vi "flashcard draw ui.vi"(0 "Color":refnum<vi>, 1 "stop":refnum<vi>, 2 "Array Info":u16[][](array[ring]) items=["Black", "White", "Orange", "Red", "Blue", "Green", "Disabled"], 3 "Cursor Size":refnum<vi>, 4 "Stunt":refnum<vi>, 5 "Flashcard Array":refnum<vi>) -> ()   [LabVIEW 2019, in "flashcards.lvlib"]
uses:
  flashcards.lvlib
  flashcards.llb/ctl_flashcard.ctl
  Colors.ctl
panel:
  in  "Pic Ring":T1
  in  "stop":bool
  out "Array":T1[][](array[typedef])=[[0, 0, 0, 0, 0, 0, 0, 0, 0, 0, 0], [0, 0, 0, 0, 0, 0, 0, 0, 0, 0, 0], [0, 0, 0, 0, 0, 0, 0, 0, 0, 0, 0], [0, 0, 0, 0, 0, 0, 0, 0, 0, 0, 0], [0, 0, 0, 0, 0, 0, 0, 0, 0, 0, 0], [0, 0, 0, 0, 0, 0, 0, 0, 0, 0, 0], [0, 0, 0, 0, 0, 0, 0, 0, 0, 0, 0], [0, 0, 0, 0, 0, 0, 0, 0, 0, 0, 0], [0, 0, 0, 0, 0, 0, 0, 0, 0, 0, 0], [0, 0, 0, 0, 0, 0, 0, 0, 0, 0, 0], [0, 0, 0, 0, 0, 0, 0, 0, 0, 0, 2]]
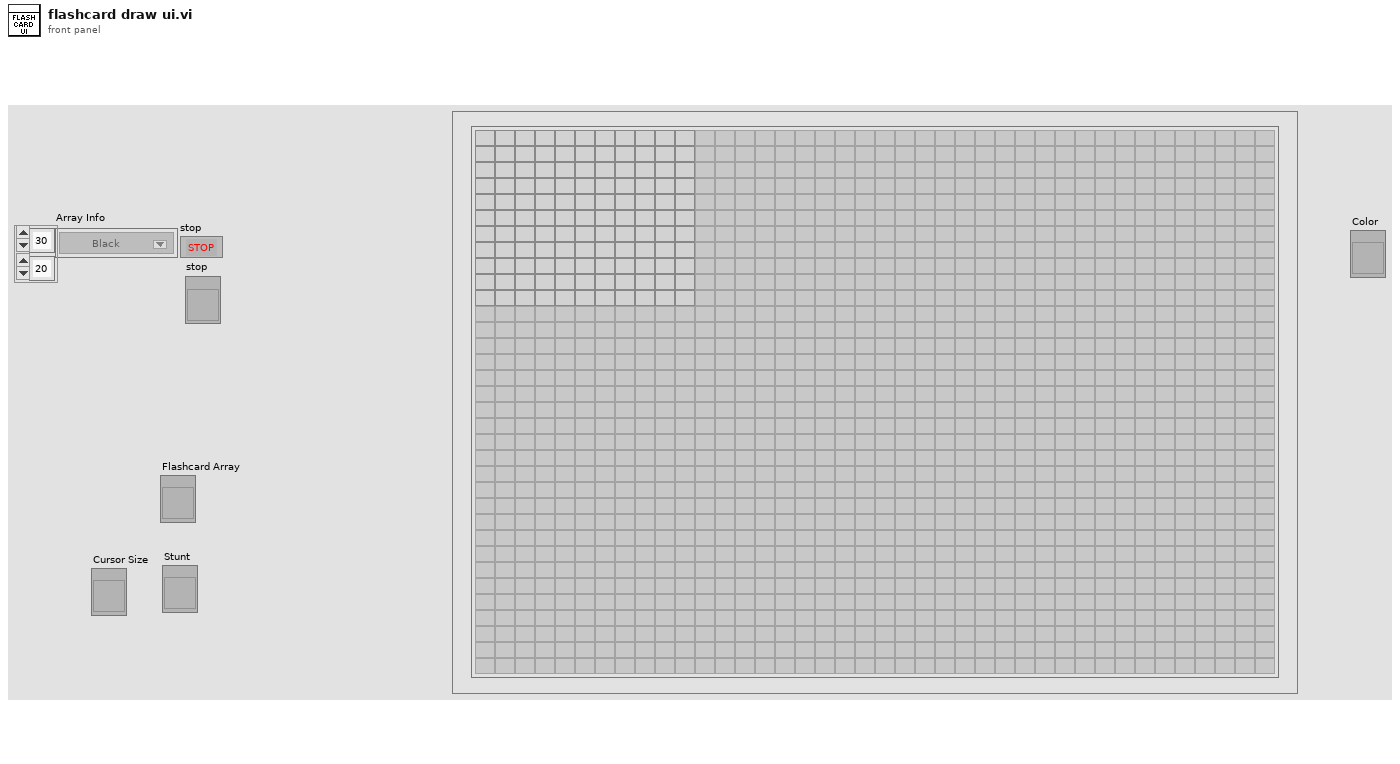
[diagram p1: front panel]
types:
  T1 = typedef "flashcards.lvlib/ctl_flashcard.ctl" = u16
  T2 = typedef "LVPositionTypeDef.ctl" = cluster{"Left":i32, "Top":i32}
  T3 = typedef "LVBoundsTypeDef.ctl" = cluster{"Width":u32, "Height":u32}
  T4 = typedef "LVPoint32TypeDef.ctl" = cluster{"Horizontal":i32, "Vertical":i32}
  T5 = typedef "Colors.ctl" = enum16{"Black", "White", "Orange", "Red", "Blue", "Green", "None"}
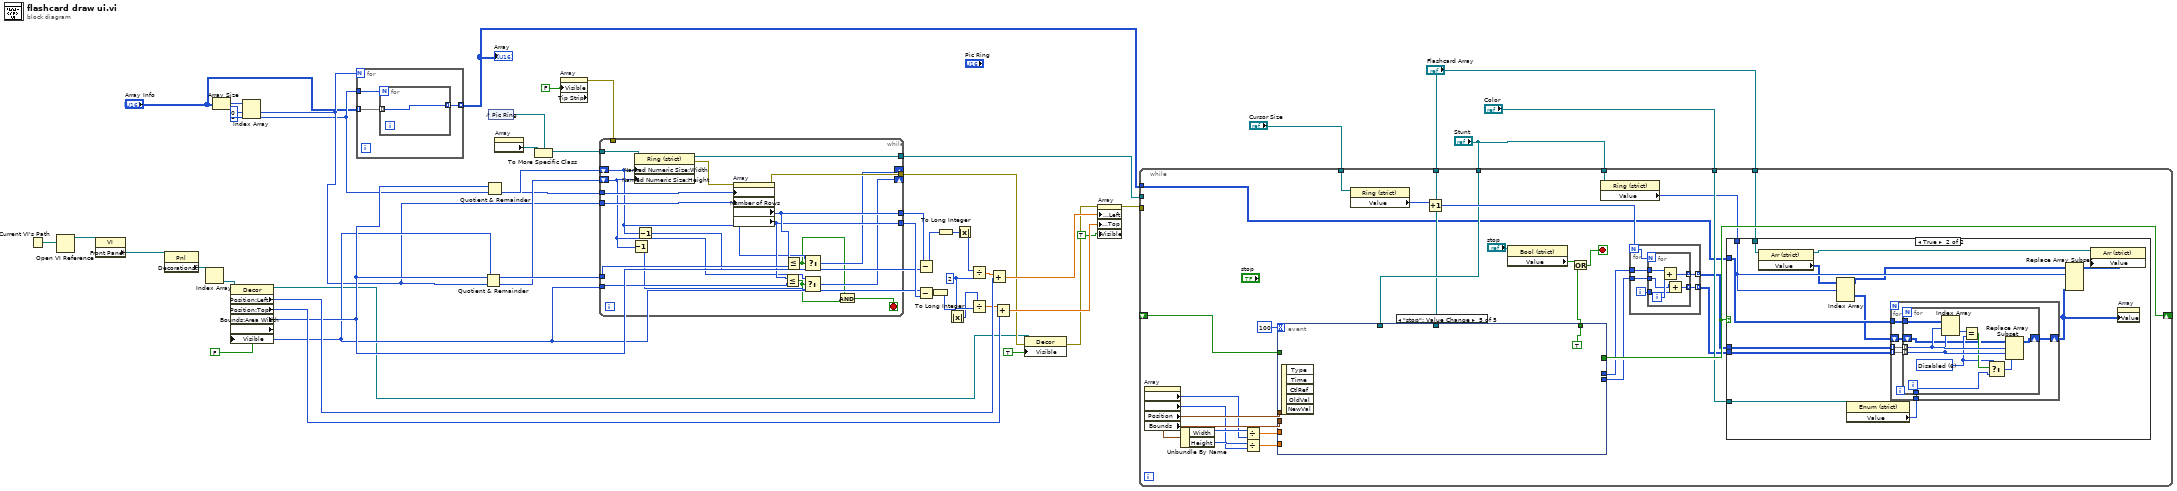
[diagram p0: block diagram]
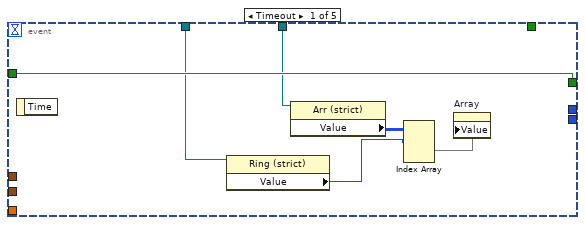
[diagram p3: hidden frame]
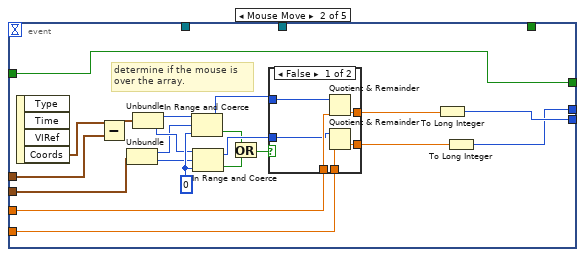
[diagram p4: hidden frame]
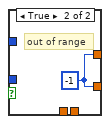
[diagram p5: hidden frame]
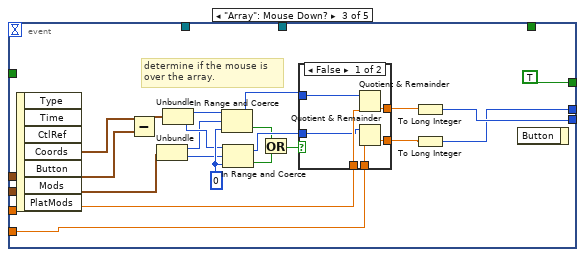
[diagram p6: hidden frame]
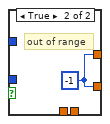
[diagram p7: hidden frame]
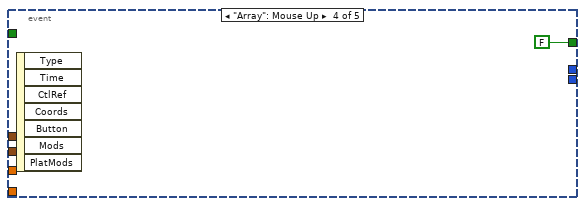
[diagram p8: hidden frame]
diagram:
  w39 = u32 2 ("y")
  n1 = Current VI's Path() -> (path=w43:path)
  n2 = Open VI Reference(vi path=w43) -> (vi reference=w44:refnum<vi>)  [unwired: 5 in, 1 out]
  n3 = property class="VI"(reference=w44) -> ("Front Panel"=w42:refnum<vi>)  [unwired: 1 in, 2 out]
  n4 = property class="Pnl"(reference=w42) -> ("Decorations[]"=w41:refnum<vi>[])  [unwired: 1 in, 2 out]
  n5 = Index Array(array=w41) -> (element=w40:refnum<vi>)  [unwired: 1 in]
  n6 = Array Size(array="Array Info") -> (size(s)=w11:i32[])
  n7 = property class="Decor"(reference=w40, "Visible"=FALSE) -> (reference out=w12:refnum<vi>, "Position:Left"=w37:i32, "Position:Top"=w35:i32, "Bounds:Area Width"=w23:u32, "Bounds:Area Height"=w22:u32)  [unwired: 1 in, 1 out]
  n8 = Index Array(array=w11, index #1=0 ("index"), index #2=1 ("index")) -> (element #1=w8:i32, element #2=w7:i32)
  n9 = for {
    N: w8 -> [_]
    tunnel: w7 -> [w51]
    tunnel: [w50] -> w2 mode=indexing
    tunnel: "Array Info" -> [w49] mode=indexing
    n10 = for {
      N: w51 -> [_]
      tunnel: [w52] -> w50 mode=indexing
      tunnel: w49 -> [w52] mode=indexing
    }
  }
  "Array" <- w2
  n11 = Quotient & Remainder(x=w22, y=w8) -> (floor(x/y)=w20:u32)  [unwired: 1 out]
  n12 = Quotient & Remainder(x=w23, y=w7) -> (floor(x/y)=w21:u32)  [unwired: 1 out]
  n13 = control-ref of="Pic Ring"() -> (w47:refnum<vi>)
  n14 = property on="Array" class="Arr (strict)"() -> ("Array Element"=w48:refnum<vi>)  [unwired: 2 in, 2 out]
  n15 = To More Specific Class(target class=w47, reference=w48) -> (specific class reference=w46:refnum<vi>)  [unwired: 1 in, 1 out]
  n16 = property on="Array" class="Arr (strict)" props=["Visible", "Tip Strip"]("Visible"=FALSE) -> (error out=w18:errorcluster)  [unwired: 2 in, 2 out]
  n17 = while {
    tunnel: w46 -> [w71]
    tunnel: [w70] -> w45
    tunnel: w7 -> [w68]
    tunnel: w8 -> [w67]
    tunnel: [w66] -> w15
    tunnel: [w65] -> w25
    tunnel: [w63] -> w24
    tunnel: w23 -> [w64]
    tunnel: w22 -> [w62]
    shift-right: [w56] -> _
    shift-left: w21 -> [w60]
    shift-right: [w57] -> _
    shift-left: w20 -> [w58]
    tunnel: w18 -> [_]
    stop <- w53 stop-if-true
    n18 = Decrement(x=w58) -> (x-1=w59:u32)
    n19 = property class="Ring (strict)"(reference=w71, "Named Numeric Size:Width"=w60, "Named Numeric Size:Height"=w58) -> (reference out=w70:refnum<vi>, error out=w69:errorcluster)  [unwired: 1 in]
    n20 = Decrement(x=w60) -> (x-1=w61:u32)
    n21 = property on="Array" class="Arr (strict)"(error in=w69, "Number of Columns"=w68, "Number of Rows"=w67) -> (error out=w66:errorcluster, "Bounds:Area Width"=w65:u32, "Bounds:Area Height"=w63:u32)  [unwired: 1 in, 1 out]
    n22 = Less Or Equal?(x=w63, y=w62) -> (x <= y?=w54:bool)
    n23 = Less Or Equal?(x=w65, y=w64) -> (x <= y?=w55:bool)
    n24 = Select(t=w58, s=w54, f=w59) -> (s? t:f=w57:u32)
    n25 = Select(t=w60, s=w55, f=w61) -> (s? t:f=w56:u32)
    n26 = And(x=w55, y=w54) -> (x .and. y?=w53:bool)
  }
  n27 = Subtract(x=w25, y=w23) -> (x-y=w31:u32)
  n28 = Subtract(x=w22, y=w24) -> (x-y=w28:u32)
  n29 = To Long Integer(number=w28) -> (32bit integer=w27:i32)
  n30 = To Long Integer(number=w31) -> (32bit integer=w30:i32)
  n31 = Absolute Value(x=w27) -> (abs(x)=w26:i32)
  n32 = Absolute Value(x=w30) -> (abs(x)=w29:i32)
  n33 = Divide(x=w29, y=w39) -> (x/y=w38:dbl)
  n34 = Divide(x=w26, y=w39) -> (x/y=w36:dbl)
  n35 = Add(x=w38, y=w37) -> (x+y=w33:dbl)
  n36 = Add(x=w36, y=w35) -> (x+y=w32:dbl)
  n37 = property class="Decor"(reference=w12, error in=w15, "Visible"=TRUE) -> (error out=w14:errorcluster)  [unwired: 1 out]
  n38 = property on="Array" class="Arr (strict)"(error in=w14, "Position:Left"=w33, "Position:Top"=w32, "Visible"=TRUE) -> (error out=w34:errorcluster)  [unwired: 1 in, 1 out]
  n39 = while {
    shift-right: [w92] -> _
    shift-left: _ -> [w91]
    tunnel: w45 -> [_]
    tunnel: w34 -> [_]
    tunnel: "Color" -> [w90]
    tunnel: "Cursor Size" -> [w89]
    tunnel: "Stunt" -> [w82]
    tunnel: "Stunt" -> [w79]
    tunnel: "Flashcard Array" -> [w78]
    tunnel: w2 -> [w77]
    tunnel: "Flashcard Array" -> [w76]
    stop <- w72 stop-if-true
    n40 = property on="Array" class="Arr (strict)"() -> ("Number of Columns"=w94:u32, "Number of Rows"=w93:u32, "Position"=w100:T2, "Bounds"=w99:T3)  [unwired: 2 in, 2 out]
    n41 = Unbundle By Name(w99) -> ("Width"=w97:u32, "Height"=w98:u32)
    n42 = Divide(x=w97, y=w94) -> (x/y=w96:dbl)
    n43 = Divide(x=w98, y=w93) -> (x/y=w95:dbl)
    n44 = event shown="[4] \"stop\": Value Change" {
      selector: _ -> [_ _ _ _ _]
      dyn-events: _ -> [_ _ _ _ _]
      timeout: 100 -> [_ _ _ _ _]
      tunnel: w100 -> [_ w155 w181 _ _]
      tunnel: w99 -> [_ w154 w182 _ _]
      tunnel: w96 -> [_ w153 w183 _ _]
      tunnel: w95 -> [_ w152 w184 _ _]
      tunnel: [_ _ _ _ TRUE] -> w73
      tunnel: [_ w147 w175 _ _] -> w86
      tunnel: [_ w148 w176 _ _] -> w85
      tunnel: [w146 w151 TRUE FALSE _] -> w92
      tunnel: w91 -> [w146 w151 _ _ _]
      tunnel: w79 -> [w145 _ _ _ _]
      tunnel: w78 -> [w144 _ _ _ _]
      event Timeout {
        n45 = event-data() -> ()  [unwired: 1 in, 1 out]
        n46 = property class="Ring (strict)"(reference=w145) -> ("Value"=w142:u16)  [unwired: 1 in, 2 out]
        n47 = property class="Arr (strict)"(reference=w144) -> ("Value"=w143:u16[][][])  [unwired: 1 in, 2 out]
        n48 = Index Array(array=w143, index (dim 0)=w142) -> (element=w141:u16[][])  [unwired: 2 in]
        n49 = property on="Array" class="Arr (strict)"("Value"=w141) -> ()  [unwired: 2 in, 2 out]
      }
      event Mouse Move {
        w162 = 0
        # "determine if the mouse is over the array."
        n50 = event-data() -> ("Coords"=w156:T4)  [unwired: 1 in, 3 out]
        n51 = Subtract(x=w156, y=w155) -> (x-y=w157:T4)
        n52 = Unbundle(w154) -> ("Width"=w159:u32, "Height"=w161:u32)
        n53 = Unbundle(w157) -> ("Horizontal"=w158:i32, "Vertical"=w160:i32)
        n54 = In Range and Coerce(upper limit=w158, x=w159, lower limit=w162) -> (coerced(x)=w166:u32, In Range?=w164:bool)
        n55 = In Range and Coerce(upper limit=w160, x=w161, lower limit=w162) -> (coerced(x)=w167:u32, In Range?=w163:bool)
        n56 = Or(x=w164, y=w163) -> (x .or. y?=w165:bool)
        n57 = case shown="False" w165 {
          tunnel: [w173 w174] -> w150
          tunnel: [w172 w174] -> w149
          tunnel: w153 -> [w171 _]
          tunnel: w152 -> [w170 _]
          tunnel: w166 -> [w169 _]
          tunnel: w167 -> [w168 _]
          frame False {
            n58 = Quotient & Remainder(x=w169, y=w171) -> (floor(x/y)=w173:dbl)  [unwired: 1 out]
            n59 = Quotient & Remainder(x=w168, y=w170) -> (floor(x/y)=w172:dbl)  [unwired: 1 out]
          }
          frame True {
            w174 = -1
            # "out of range"
          }
        }
        n60 = To Long Integer(number=w150) -> (32bit integer=w148:i32)
        n61 = To Long Integer(number=w149) -> (32bit integer=w147:i32)
      }
      event "Array": Mouse Down? {
        w190 = 0
        # "determine if the mouse is over the array."
        n62 = event-data() -> ("Coords"=w180:T4)  [unwired: 1 in, 6 out]
        n63 = Subtract(x=w180, y=w181) -> (x-y=w185:T4)
        n64 = Unbundle(w182) -> ("Width"=w187:u32, "Height"=w189:u32)
        n65 = Unbundle(w185) -> ("Horizontal"=w186:i32, "Vertical"=w188:i32)
        n66 = In Range and Coerce(upper limit=w186, x=w187, lower limit=w190) -> (coerced(x)=w194:u32, In Range?=w192:bool)
        n67 = In Range and Coerce(upper limit=w188, x=w189, lower limit=w190) -> (coerced(x)=w195:u32, In Range?=w191:bool)
        n68 = Or(x=w192, y=w191) -> (x .or. y?=w193:bool)
        n69 = case shown="False" w193 {
          tunnel: [w201 w202] -> w179
          tunnel: [w200 w202] -> w178
          tunnel: w183 -> [w199 _]
          tunnel: w184 -> [w198 _]
          tunnel: w194 -> [w197 _]
          tunnel: w195 -> [w196 _]
          frame False {
            n70 = Quotient & Remainder(x=w197, y=w199) -> (floor(x/y)=w201:dbl)  [unwired: 1 out]
            n71 = Quotient & Remainder(x=w196, y=w198) -> (floor(x/y)=w200:dbl)  [unwired: 1 out]
          }
          frame True {
            w202 = -1
            # "out of range"
          }
        }
        n72 = To Long Integer(number=w179) -> (32bit integer=w176:i32)
        n73 = To Long Integer(number=w178) -> (32bit integer=w175:i32)
        n74 = event-data() -> ()  [unwired: 2 in, 1 out]
      }
      event "Array": Mouse Up {
        n75 = event-data() -> ()  [unwired: 1 in, 7 out]
      }
      event "stop": Value Change {
        n76 = event-data() -> ()  [unwired: 1 in, 5 out]
      }
    }
    n77 = property class="Ring (strict)"(reference=w89) -> ("Value"=w88:u16)  [unwired: 1 in, 2 out]
    n78 = Increment(x=w88) -> (x+1=w87:u16)
    n79 = property class="Bool (strict)"(reference="stop") -> ("Value"=w74:bool)  [unwired: 1 in, 2 out]
    n80 = Or(x=w74, y=w73) -> (x .or. y?=w72:bool)
    n81 = property class="Ring (strict)"(reference=w82) -> ("Value"=w81:u16)  [unwired: 1 in, 2 out]
    n82 = for {
      N: w87 -> [w101]
      tunnel: w86 -> [w106]
      tunnel: w85 -> [w105]
      tunnel: [w103] -> w83 mode=indexing
      tunnel: [w102] -> w84 mode=indexing
      i -> [w104]
      n83 = for {
        N: w101 -> [_]
        tunnel: w106 -> [w112]
        tunnel: w105 -> [w110]
        tunnel: w104 -> [w109]
        tunnel: [w108] -> w103 mode=indexing
        tunnel: [w107] -> w102 mode=indexing
        i -> [w111]
        n84 = Add(x=w112, y=w111) -> (x+y=w107:i32)
        n85 = Add(x=w110, y=w109) -> (x+y=w108:i32)
      }
    }
    n86 = case shown="True" w92 {
      tunnel: w90 -> [_ w124]
      tunnel: w84 -> [_ w122]
      tunnel: w83 -> [_ w121]
      tunnel: w81 -> [_ w120]
      tunnel: w77 -> [_ w118]
      tunnel: w76 -> [_ w117]
      frame False {
      }
      frame True {
        n87 = property class="Arr (strict)"(reference=w117) -> (reference out=w113:refnum<vi>, "Value"=w116:u16[][][])  [unwired: 1 in, 1 out]
        n88 = Index Array(array=w116, index (dim 0)=w120) -> (element=w115:u16[][])  [unwired: 2 in]
        n89 = property class="Enum (strict)"(reference=w124) -> ("Value"=w123:T5)  [unwired: 1 in, 2 out]
        n90 = for {
          tunnel: w122 -> [w130] mode=indexing
          tunnel: w121 -> [w129] mode=indexing
          tunnel: w123 -> [w128]
          shift-right: [w125] -> w119
          shift-left: w115 -> [w127]
          tunnel: w118 -> [w126]
          n91 = for {
            tunnel: w130 -> [w140] mode=indexing
            tunnel: w129 -> [w139] mode=indexing
            tunnel: w128 -> [w137]
            shift-right: [w131] -> w125
            shift-left: w127 -> [w133]
            tunnel: w126 -> [w132]
            w135 = u16 6 items=["Black", "White", "Orange", "Red", "Blue", "Green", "Disabled"] ("Color")
            n92 = Index Array(array=w132, index (row)=w140, index (col)=w139) -> (element=w138:u16)
            n93 = Equal?(x=w138, y=w135) -> (x = y?=w136:bool)
            n94 = Select(t=w135, s=w136, f=w137) -> (s? t:f=w134:u16)
            n95 = Replace Array Subset(array=w133, new element=w134, index (row)=w140, index (col)=w139) -> (w131:u16[][])
          }
        }
        n96 = Replace Array Subset(array=w116, new element=w119, index (dim 0)=w120) -> (w114:u16[][][])  [unwired: 2 in]
        n97 = property class="Arr (strict)"(reference=w113, "Value"=w114) -> ()  [unwired: 1 in, 2 out]
        n98 = property on="Array" class="Arr (strict)"("Value"=w119) -> ()  [unwired: 2 in, 2 out]
      }
    }
  }
